vi "Stop Server.vi"(8 "error in (no error)":errorcluster, 11 "Server in":refnum<class "Server.lvclass">) -> (0 "error out":errorcluster, 3 "Server out":refnum<class "Server.lvclass">)   [LabVIEW 2013, in "MQTT Server.lvlib" / "Server.lvclass"]
uses:
  Server.lvclass
  Server.lvclass/Server.ctl
  ConnectionHandler/TCPConnectionHandler.lvclass
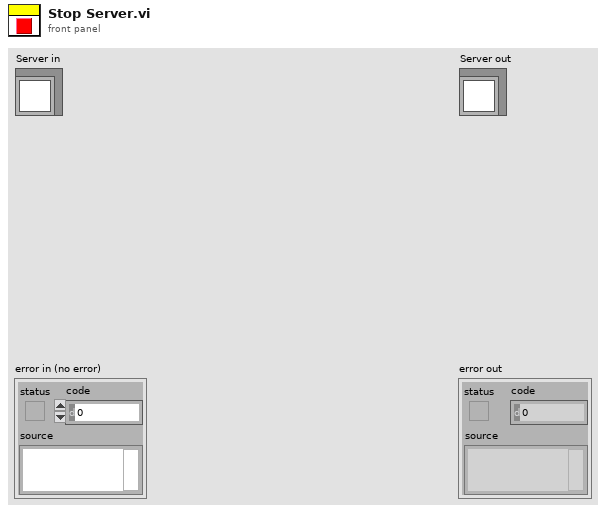
[diagram p1: front panel]
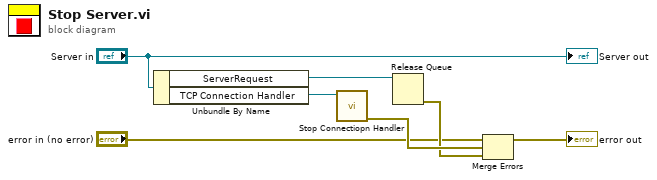
[diagram p0: block diagram]
diagram:
  n1 = Unbundle By Name("Server in") -> ("ServerRequest"=w6:refnum<queue>, "TCP Connection Handler"=w5:refnum<class "TCPConnectionHandler.lvclass">)
  n2 = call "Stop Connectiopn Handler.vi"("TCPConnectionHandler in"=w5) -> ("error out"=w4:errorcluster)  [unwired: 9 in, 1 out]
  n3 = Release Queue(queue=w6) -> (error out=w3:errorcluster)  [unwired: 2 in, 2 out]
  n4 = Merge Errors("error in (no error)", w4, w3) -> (→"error out":errorcluster)
  "Server out" <- "Server in"
